vi "Get Channel Data Type.vi"(8 "error in":errorcluster, 11 "Channel in":refnum<k20>) -> (0 "error out":errorcluster, 1 "Units":string, 2 "Data Type":string, 3 "Channel out":refnum<k20>)   [LabVIEW 2011, in "Engine Sim System Explorer.lvlib" / "Engine Sim File Interface.lvlib"]
uses:
  Engine Sim File Interface.lvlib
  <vilib>/Platform/storage/Storage.llb/Get Property (Enum).vi
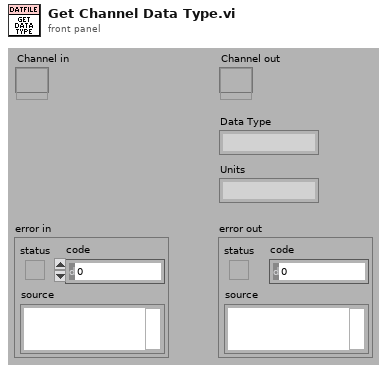
[diagram p1: front panel]
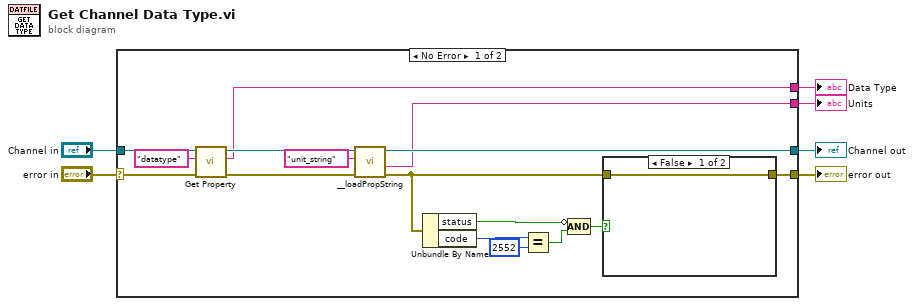
[diagram p0: block diagram]
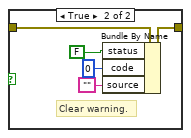
[diagram p2: hidden frame]
diagram:
  n1 = case shown="No Error" "error in" {
    selector: "error in" -> [w16 w29]
    tunnel: "Channel in" -> [w20 w30]
    tunnel: [w17 w30] -> w5
    tunnel: [w11 _] -> w3
    tunnel: [w10 _] -> w2
    tunnel: [w8 w29] -> w1
    frame No Error {
      n2 = call-poly <vilib>:"Get Property.vi"("error in (no error)"=w16, "Property name"="datatype" ("Data type"), "storage refnum"=w20) -> ("error out"=w22:errorcluster, "String"=w10:string, "storage refnum out"=w21:refnum<k20>)  [unwired: 6 out]
      n3 = call <vilib>:"__loadPropString.vi"("error in (no error)"=w22, "Property name"="unit_string", "storage refnum"=w21) -> ("error out"=w7:errorcluster, "Value"=w11:string, "dup storage refnum"=w17:refnum<k20>)  [unwired: 6 in]
      n4 = Unbundle By Name(w7) -> ("status"=w13:bool, "code"=w15:i32)
      n5 = Equal?(x=w15, y=2552) -> (x = y?=w12:bool)
      n6 = Compound Arithmetic op=AND(invert w13, w12) -> (w9:bool)
      n7 = case shown="False" w9 {
        tunnel: [w23 w27] -> w8
        tunnel: w7 -> [w23 w28]
        frame False {
        }
        frame True {
          # "Clear warning."
          n8 = Bundle By Name(cluster=w28, "status"=FALSE, "code"=0, "source"="") -> (w27:errorcluster)
        }
      }
    }
    frame Error {
    }
  }
  "error out" <- w1
  "Channel out" <- w5
  "Data Type" <- w2
  "Units" <- w3
